vi "Get Bucket Website Configuration.vi"(4 "Region":T1, 8 "error in (no error)":errorcluster, 9 "Bucket":string) -> (0 "error out":errorcluster, 3 "WebsiteConfiguration":T2)   [LabVIEW 2015, in "LV Interface for Amazon S3.lvlib"]
doc: "This operation <B>returns the website configuration</B>. This operation <B>requires the S3:GetBucketWebsite permission</B>. By default, only the bucket owner can read the bucket website configuration. Bucket <B>owners can allow other users to read the website configuration by</B> writing a bucket policy <B>granting them the S3:GetBucketWebsite permission</B>."
uses:
  LV Interface for Amazon S3.lvlib
  Typedefs/AMZ_S3_API_WebsiteConfiguration.ctl
  Typedefs/AMZ_S3_LocationConstraint.ctl
  XML Parser/XML Parser.lvlib
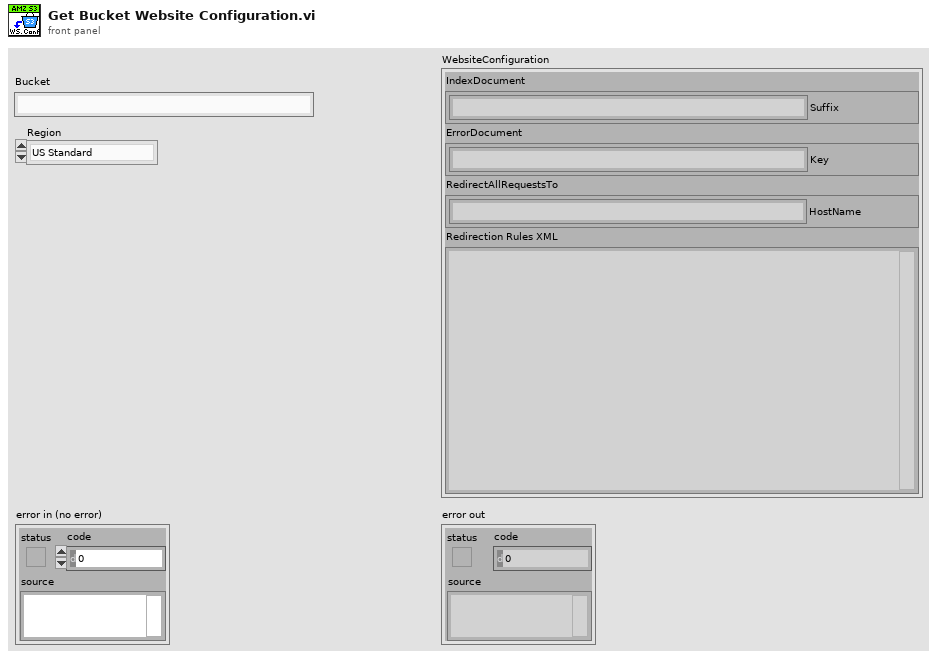
[diagram p1: front panel]
types:
  T1 = typedef "LV Interface for Amazon S3.lvlib/AMZ_S3_LocationConstraint.ctl" = enum16{"US Standard", "us-east-2", "us-west-1", "us-west-2", "ap-northeast-1", "ap-northeast-2", "ap-southeast-1", "ap-southeast-2", "ca-central-1", "eu-central-1", "eu-west-1", "eu-west-2", "sa-east-1"}
  T2 = typedef "LV Interface for Amazon S3.lvlib/AMZ_S3_API_WebsiteConfiguration.ctl" = cluster{"IndexDocument":cluster{"Suffix":string}, "ErrorDocument":cluster{"Key":string}, "RedirectAllRequestsTo":cluster{"HostName":string}, "Redirection Rules XML":string}
  T3 = typedef "LV Interface for Amazon S3.lvlib/AMZ_S3_Call Results.ctl" = enum16{"Success", "UndefinedError", "AccessDenied", "AccountProblem", "AmbiguousGrantByEmailAddress", "BadDigest", "BucketAlreadyExists", "BucketAlreadyOwnedByYou", "BucketNotEmpty", "CredentialsNotSupported", "CrossLocationLoggingProhibited", "EntityTooSmall", "EntityTooLarge", "ExpiredToken", "IllegalVersioningConfigurationException", "IncompleteBody", "IncorrectNumberOfFilesInPostRequest", "InlineDataTooLarge", "InternalError", "InvalidAccessKeyId", "InvalidAddressingHeader", "InvalidArgument", "InvalidBucketName", "InvalidDigest", "InvalidLocationConstraint", "InvalidPart", "InvalidPartOrder", "InvalidPayer", "InvalidPolicyDocument", "InvalidRange", "InvalidSecurity", "InvalidSOAPRequest", "InvalidStorageClass", "InvalidTargetBucketForLogging", "InvalidToken", "InvalidURI", "KeyTooLong", "MalformedACLError", "MalformedPOSTRequest", "MalformedXML", "MaxMessageLengthExceeded", "MaxPostPreDataLengthExceededError", "MetadataTooLarge", "MethodNotAllowed", "MissingAttachment", "MissingContentLength", "MissingRequestBodyError", "MissingSecurityElement", "MissingSecurityHeader", "NoLoggingStatusForKey", "NoSuchBucket", "NoSuchKey", "NoSuchUpload", "NoSuchVersion", "NotImplemented", "NotSignedUp", "OperationAborted", "PermanentRedirect", "PreconditionFailed", "Redirect", "RequestIsNotMultiPartContent", "RequestTimeout", "RequestTimeTooSkewed", "RequestTorrentOfBucketError", "SignatureDoesNotMatch", "SlowDown", "TemporaryRedirect", "TokenRefreshRequired", "TooManyBuckets", "UnexpectedContent", "UnresolvableGrantByEmailAddress", "UserKeyMustBeSpecified", "LabVIEWError"}
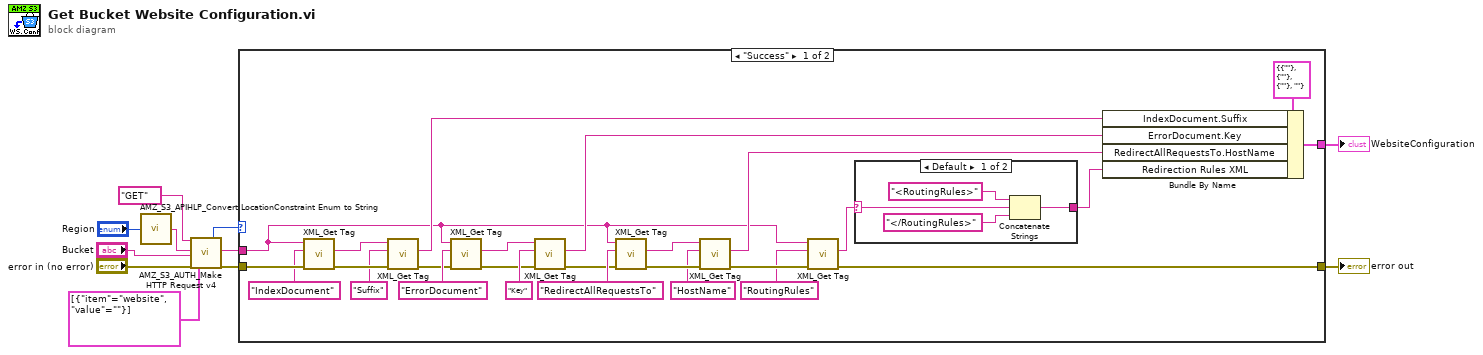
[diagram p0: block diagram]
diagram:
  n1 = call "AMZ_S3_APIHLP_Convert LocationConstraint Enum to String.vi"("Location"="Region") -> ("Location String"=w1:string)  [unwired: 4 in]
  n2 = call "AMZ_S3_AUTH_Make HTTP Request v4.vi"("HTTP-Verb"="GET", "Region"=w1, "Bucket"="Bucket", "error in"="error in (no error)", "request parameters"=cluster{"item":string, "value":string}[] [{"item"="website", "value"=""}]) -> ("Call Result"=w5:T3, "response body"=w4:string, "error out"=w8:errorcluster)  [unwired: 11 in, 1 out]
  n3 = case shown="\"Success\"" w5 {
    tunnel: w8 -> [w37 w42]
    tunnel: w4 -> [w14 _]
    tunnel: [w35 _] -> w11
    tunnel: [w16 w42] -> w10
    frame "Success" {
      n4 = call "XML_Get Tag.vi"("error in (no error)"=w37, "Tag name"="IndexDocument", "XML String in"=w14) -> ("error out"=w33:errorcluster, "Tag value"=w32:string)  [unwired: 4 in, 3 out]
      n5 = call "XML_Get Tag.vi"("error in (no error)"=w33, "Tag name"="Suffix", "XML String in"=w32) -> ("error out"=w25:errorcluster, "Tag value"=w30:string)  [unwired: 4 in, 3 out]
      n6 = call "XML_Get Tag.vi"("error in (no error)"=w25, "Tag name"="ErrorDocument", "XML String in"=w14) -> ("error out"=w27:errorcluster, "Tag value"=w28:string)  [unwired: 4 in, 3 out]
      n7 = call "XML_Get Tag.vi"("error in (no error)"=w27, "Tag name"="Key", "XML String in"=w28) -> ("error out"=w19:errorcluster, "Tag value"=w24:string)  [unwired: 4 in, 3 out]
      n8 = call "XML_Get Tag.vi"("error in (no error)"=w19, "Tag name"="RedirectAllRequestsTo", "XML String in"=w14) -> ("error out"=w22:errorcluster, "Tag value"=w21:string)  [unwired: 4 in, 3 out]
      n9 = call "XML_Get Tag.vi"("error in (no error)"=w22, "Tag name"="HostName", "XML String in"=w21) -> ("error out"=w17:errorcluster, "Tag value"=w18:string)  [unwired: 4 in, 3 out]
      n10 = call "XML_Get Tag.vi"("error in (no error)"=w17, "Tag name"="RoutingRules", "XML String in"=w14) -> ("error out"=w16:errorcluster, "Tag value"=w13:string)  [unwired: 4 in, 3 out]
      n11 = case shown="Default" w13 {
        selector: w13 -> [w41 _]
        tunnel: [w40 _] -> w12
        frame Default {
          n12 = Concatenate Strings("<RoutingRules>", w41, "</RoutingRules>") -> (w40:string)
        }
        frame "" {
        }
      }
      n13 = Bundle By Name(cluster=T2 {"IndexDocument"={"Suffix"=""}, "ErrorDocument"={"Key"=""}, "RedirectAllRequestsTo"={"HostName"=""}, "Redirection Rules XML"=""} ("WebsiteConfiguration"), "IndexDocument.Suffix"=w30, "ErrorDocument.Key"=w24, "RedirectAllRequestsTo.HostName"=w18, "Redirection Rules XML"=w12) -> (w35:T2)
    }
    frame Default {
    }
  }
  "error out" <- w10
  "WebsiteConfiguration" <- w11
